vi "Fetch Trigger Times.vi"(8 "error in (no error)":errorcluster, 9 "Timeout (10000 ms)":u32=10000, 10 "Source (0: Channel 1)":u16(ring) items=["Channel 1", "Channel 2", "Channel 3", "Channel 4", "Memory 1", "Memory 2", "Memory 3", "Memory 4", "Function 1", "Function 2", "Function 3", "Function 4", "Function 5", "Function 6", "Function 7", "Function 8"], 11 "VISA resource name":refnum<visa-resource-name>) -> (0 "error out":errorcluster, 1 "Trigger Offset":dbl[](array[numeric]), 2 "Trigger Time":dbl[](array[numeric]), 3 "VISA resource name out":refnum<visa-resource-name>)   [LabVIEW 2015, in "LeCroy Wave Series.lvlib"]
doc: "Gets for all segments trigger time and trigger offset.\n\nNote:\nThis optional time array is only present with SEQNCE waveforms."
uses:
  <instrlib>/LeCroy Wave Series/LeCroy Wave Series.lvlib
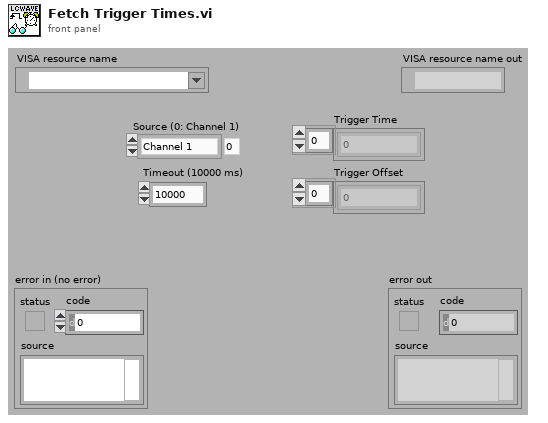
[diagram p1: front panel]
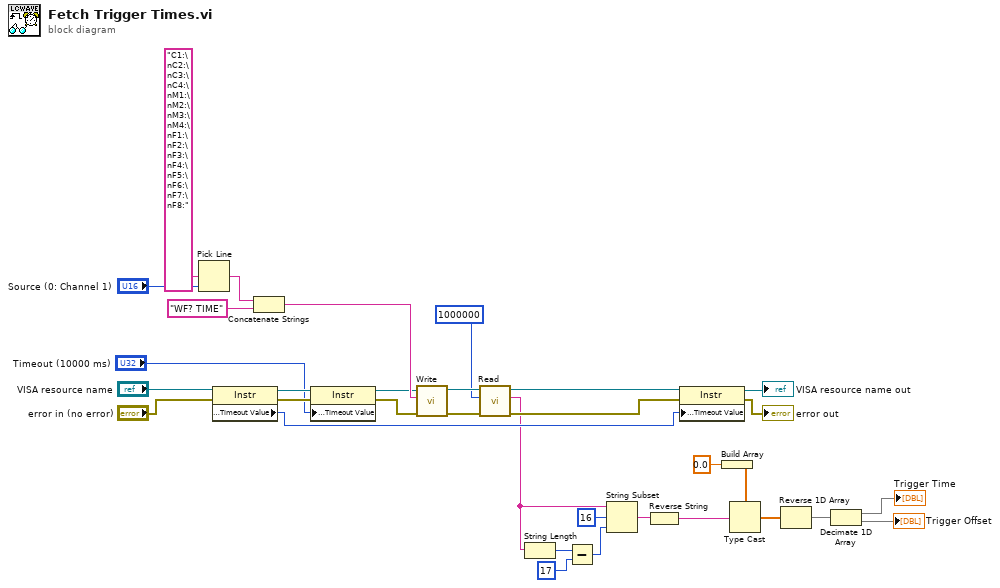
[diagram p0: block diagram]
diagram:
  n1 = Pick Line(multi-line string="C1:\nC2:\nC3:\nC4:\nM1:\nM2:\nM3:\nM4:\nF1:\nF2:\nF3:\nF4:\nF5:\nF6:\nF7:\nF8:", line index="Source (0: Channel 1)") -> (output string=w29:string)  [unwired: 1 in]
  n2 = property on="Property Node" class="Instr"(reference="VISA resource name", error in="error in (no error)") -> (reference out=w25:refnum<visa-resource-name>, error out=w24:errorcluster, "General Settings:Timeout Value"=w17:u32)
  n3 = Concatenate Strings(w29, "WF? TIME" ("write buffer")) -> (w33:string)
  n4 = property on="Property Node" class="Instr"(reference=w25, error in=w24, "General Settings:Timeout Value"="Timeout (10000 ms)") -> (reference out=w23:refnum<visa-resource-name>, error out=w22:errorcluster)
  n5 = call <instrlib>:"Write.vi"("error in (no error)"=w22, "Write Buffer"=w33, "VISA resource name"=w23) -> ("error out"=w31:errorcluster, "VISA resource name out"=w32:refnum<visa-resource-name>)  [unwired: 6 in, 1 out]
  n6 = call <instrlib>:"Read.vi"("error in (no error)"=w31, "Byte Count"=u32 1000000, "VISA resource name"=w32) -> ("error out"=w20:errorcluster, "Read Buffer"=w4:string, "VISA resource name out"=w21:refnum<visa-resource-name>)  [unwired: 5 in, 1 out]
  n7 = String Length(string=w4) -> (length=w3:i32)
  n8 = Subtract(x=w3, y=17 ("offset (0)")) -> (x-y=w1:i32)
  n9 = String Subset(string=w4, offset (0)=16, length (rest)=w1) -> (substring=w5:string)
  n10 = Reverse String(1:w5) -> (0:w7:string)
  n11 = property on="Property Node" class="Instr"(reference=w21, error in=w20, "General Settings:Timeout Value"=w17) -> (reference out=→"VISA resource name out":refnum<visa-resource-name>, error out=→"error out":errorcluster)
  n12 = Build Array(0.0) -> (w12:dbl[])
  n13 = Type Cast(type=w12, x=w7) -> (*(type *) &x=w11:dbl[])
  n14 = Reverse 1D Array(array=w11) -> (reversed array=w6:dbl[])
  n15 = Decimate 1D Array(w6) -> (→"Trigger Time":dbl[], →"Trigger Offset":dbl[])
